vi "ClustertoTagbus.vi"(8 "error in":errorcluster, 9 "index cluster":T1, 10 "cluster":T2, 11 "tag bus in":T3) -> (0 "error out":errorcluster, 3 "tag bus out":T3)   [LabVIEW 2013]
uses:
  <vilib>/NI/Tag Bus/table/data table.ctl
  Controls/SampleControl.ctl
  Controls/IndexCluster.ctl
  <vilib>/NI/Tag Bus/table/data polymorphs/write one/write Array of Double.vi
  <vilib>/NI/Tag Bus/table/data polymorphs/write one/write Boolean.vi
  <vilib>/NI/Tag Bus/table/data polymorphs/write one/write Double.vi
  <vilib>/NI/Tag Bus/table/data polymorphs/write one/write String.vi
  <vilib>/NI/Tag Bus/table/data table.lvlib
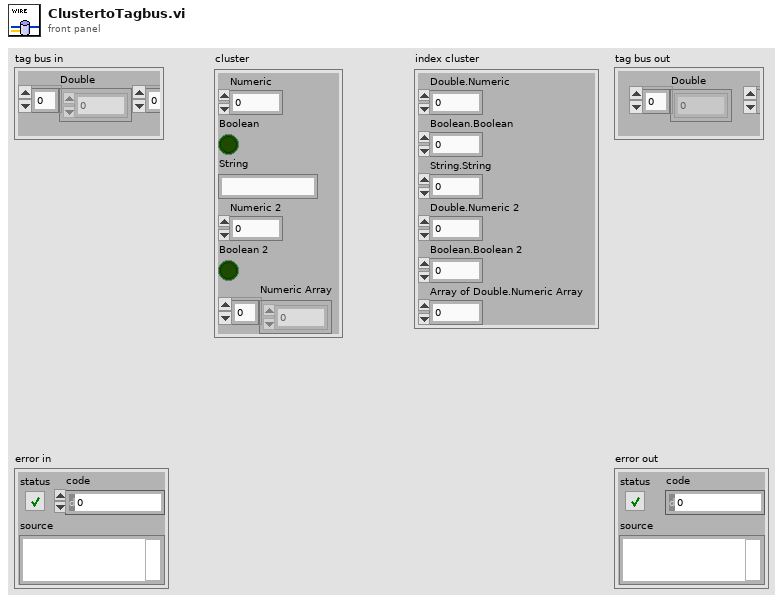
[diagram p1: front panel]
types:
  T1 = typedef "IndexCluster.ctl" = cluster{"Double.Numeric":i32, "Boolean.Boolean":i32, "String.String":i32, "Double.Numeric 2":i32, "Boolean.Boolean 2":i32, "Array of Double.Numeric Array":i32}
  T2 = typedef "SampleControl.ctl" = cluster{"Numeric":dbl, "Boolean":bool, "String":string, "Numeric 2":dbl, "Boolean 2":bool, "Numeric Array":dbl[]}
  T3 = typedef "tag bus.lvlib/data table.lvlib/data table.ctl" = cluster{"Double":dbl[], "Single":sgl[], "I64":i64[], "I32":i32[], "I16":i16[], "I8":i8[], "U64":u64[], "U32":u32[], "U16":u16[], "U8":u8[], "Boolean":bool[], "String":string[], "Array of Double":cluster{"DBL Array":dbl[]}[], "Array of Single":cluster{"SGL Array":sgl[]}[], "Array of I64":cluster{"I64 Array":i64[]}[], "Array of I32":cluster{"I32 Array":i32[]}[], "Array of I16":cluster{"I16 Array":i16[]}[], "Array of I8":cluster{"I8 Array":i8[]}[], "Array of U64":cluster{"U64 Array":u64[]}[], "Array of U32":cluster{"U32 Array":u32[]}[], "Array of U16":cluster{"U16 Array":u16[]}[], "Array of U8":cluster{"U8 Array":u8[]}[], "Array of Boolean":cluster{"Boolean Array":bool[]}[], "Array of String":cluster{"String Array":string[]}[]}
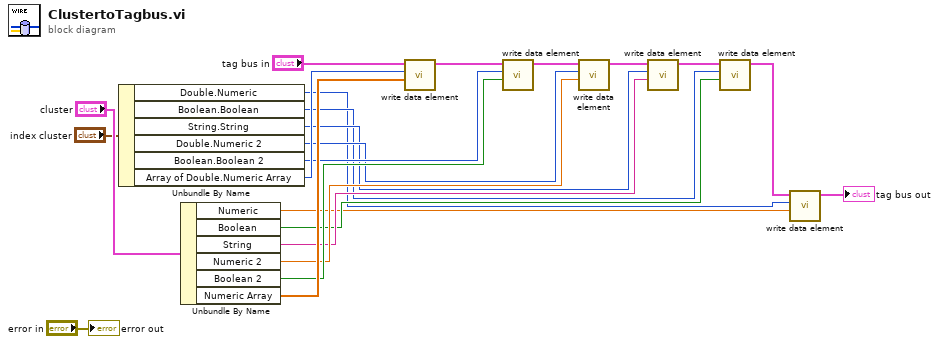
[diagram p0: block diagram]
diagram:
  n1 = Unbundle By Name("index cluster") -> ("Double.Numeric"=w5:i32, "Boolean.Boolean"=w8:i32, "String.String"=w11:i32, "Double.Numeric 2"=w14:i32, "Boolean.Boolean 2"=w17:i32, "Array of Double.Numeric Array"=w20:i32)
  n2 = Unbundle By Name("cluster") -> ("Numeric"=w4:dbl, "Boolean"=w7:bool, "String"=w10:string, "Numeric 2"=w13:dbl, "Boolean 2"=w16:bool, "Numeric Array"=w19:dbl[])
  n3 = call-poly <vilib>:"write data element.vi"("value"=w19, "index"=w20, "data table in"="tag bus in") -> ("data table out"=w15:T3)  [unwired: 8 in]
  n4 = call-poly <vilib>:"write data element.vi"("value"=w16, "index"=w17, "data table in"=w15) -> ("data table out"=w12:T3)  [unwired: 8 in]
  n5 = call-poly <vilib>:"write data element.vi"("value"=w13, "index"=w14, "data table in"=w12) -> ("data table out"=w9:T3)  [unwired: 8 in]
  n6 = call-poly <vilib>:"write data element.vi"("value"=w10, "index"=w11, "data table in"=w9) -> ("data table out"=w6:T3)  [unwired: 8 in]
  n7 = call-poly <vilib>:"write data element.vi"("value"=w7, "index"=w8, "data table in"=w6) -> ("data table out"=w3:T3)  [unwired: 8 in]
  n8 = call-poly <vilib>:"write data element.vi"("value"=w4, "index"=w5, "data table in"=w3) -> ("data table out"=→"tag bus out":T3)  [unwired: 8 in]
  "error out" <- "error in"
